vi "Initialize Inline Buffer.vi"(8 "error in (no error)":errorcluster, 9 "size":u64 format="%d bytes", 10 "address":u64 format="%016x", 11 "Framework in":refnum<class "Framework.lvclass">) -> (0 "error out":errorcluster, 3 "Framework out":refnum<class "Framework.lvclass">)   [LabVIEW 2017, in "DSF Core.lvlib" / "Framework.lvclass"]
uses:
  Framework.lvclass
  Buffer/Buffer.lvclass
  C:/Git/DSF/LabVIEW-Memory/Source/Classes/Pointer/Pointer.lvclass
  Framework.lvclass/Framework.ctl
  LabVIEW-Memory/Source/Classes/Pointer/Pointer.lvclass
  Buffers/Buffers.lvclass
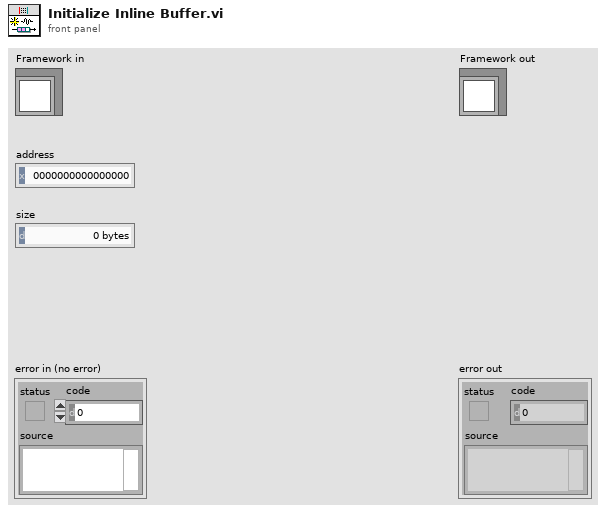
[diagram p1: front panel]
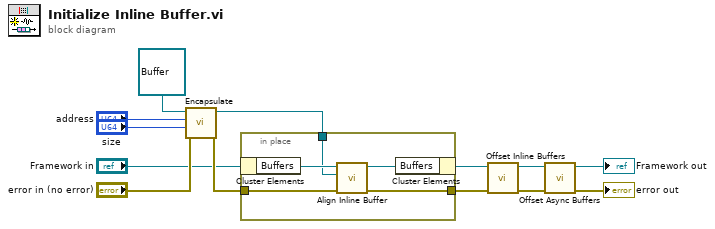
[diagram p0: block diagram]
diagram:
  n1 = call "Encapsulate.vi"("error in (no error)"="error in (no error)", "size"="size", "address"="address", "Pointer in"=refnum<class "Buffer.lvclass"> refnum ("Inline Buffer")) -> ("error out"=w6:errorcluster, "Pointer out"=w3:refnum<class "Buffer.lvclass">)  [unwired: 6 in]
  n2 = in-place {
    in-place-border: w6 -> [w15]
    in-place-border: [w16] -> w4
    in-place-border: w3 -> [w14]
    n3 = in-place-cluster #1("Framework in") -> ("Buffers"=w18:refnum<class "Buffers.lvclass">)
    n4 = call "Align Inline Buffer.vi"("error in (no error)"=w15, "base Inline Buffer"=w14, "Buffers in"=w18) -> ("error out"=w16:errorcluster, "Buffers out"=w17:refnum<class "Buffers.lvclass">)  [unwired: 7 in]
    n5 = in-place-cluster #1("Buffers"=w17) -> (w2:refnum<class "Framework.lvclass">)
  }
  n6 = call "Offset Inline Buffers.vi"("error in (no error)"=w4, "Framework in"=w2) -> ("error out"=w10:errorcluster, "Framework out"=w11:refnum<class "Framework.lvclass">)  [unwired: 8 in]
  n7 = call "Offset Async Buffers.vi"("error in (no error)"=w10, "Framework in"=w11) -> ("error out"=→"error out":errorcluster, "Framework out"=→"Framework out":refnum<class "Framework.lvclass">)  [unwired: 8 in]
